vi "MVE Get Project and Library Refnums.vi"(8 "error in (no error)":errorcluster, 10 "Full Path":string) -> (0 "error out":errorcluster, 2 "ProjectItem Refnum":refnum<vi>, 3 "Project Refnum":refnum<vi>)   [LabVIEW 2016]
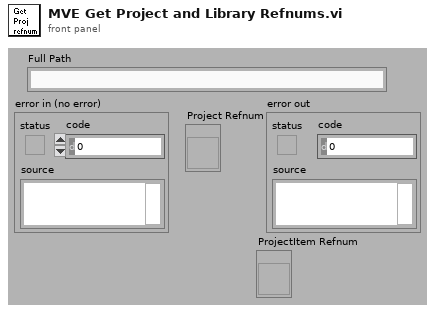
[diagram p1: front panel]
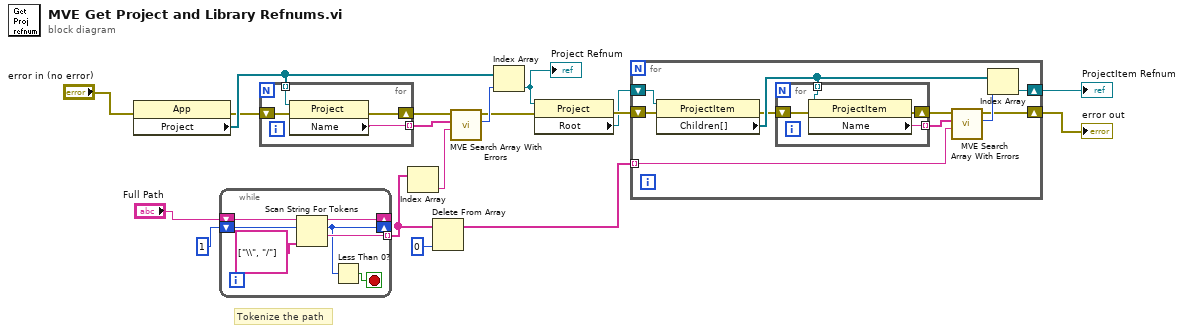
[diagram p0: block diagram]
diagram:
  # "Tokenize the path"
  n1 = property class="App"(error in="error in (no error)") -> (error out=w10:errorcluster, "Project"=w18:refnum<vi>[])  [unwired: 1 in, 1 out]
  n2 = while {
    tunnel: [w21] -> w14 mode=indexing
    shift-right: [w25] -> _
    shift-left: "Full Path" -> [w24]
    shift-right: [w19] -> _
    shift-left: 1 ("offset past token") -> [w23]
    stop <- w20 stop-if-true
    n3 = Scan String For Tokens(6:string[] ["\\", "/"] ("delimiters (\\s,\\t,\\r,\\n)"), 8:w23, 9:w24) -> (1:w21:string, 2:w19:i32, 3:w25:string)  [unwired: 3 in, 1 out]
    n4 = Less Than 0?(x=w19) -> (x < 0?=w20:bool)
  }
  n5 = for {
    tunnel: w18 -> [w29] mode=indexing
    tunnel: [w28] -> w6 mode=indexing
    shift-right: [w26] -> w7
    shift-left: w10 -> [w27]
    n6 = property class="Project"(reference=w29, error in=w27) -> (error out=w26:errorcluster, "Name"=w28:string)  [unwired: 1 out]
  }
  n7 = Index Array(array=w14) -> (element=w8:string)  [unwired: 1 in]
  n8 = Delete From Array(array=w14, index=0) -> (array with subset deleted=w5:string[])  [unwired: 1 in, 1 out]
  n9 = call <resource>:"MVE Search Array With Errors.vi"("String"=w8, "Array of Strings"=w6, "error in (no error)"=w7) -> ("index of element"=w17:i32, "error out"=w4:errorcluster)  [unwired: 7 in]
  n10 = Index Array(array=w18, index=w17) -> (element=w12:refnum<vi>)
  "Project Refnum" <- w12
  n11 = property class="Project"(reference=w12, error in=w4) -> (error out=w9:errorcluster, "Root"=w3:refnum<vi>)  [unwired: 1 out]
  n12 = for {
    tunnel: w5 -> [w32] mode=indexing
    shift-right: [w37] -> w1
    shift-left: w3 -> [w39]
    shift-right: [w33] -> w2
    shift-left: w9 -> [w35]
    n13 = property class="ProjectItem"(reference=w39, error in=w35) -> (error out=w34:errorcluster, "Children[]"=w38:refnum<vi>[])  [unwired: 1 out]
    n14 = for {
      tunnel: w38 -> [w43] mode=indexing
      tunnel: [w42] -> w31 mode=indexing
      shift-right: [w40] -> w30
      shift-left: w34 -> [w41]
      n15 = property class="ProjectItem"(reference=w43, error in=w41) -> (error out=w40:errorcluster, "Name"=w42:string)  [unwired: 1 out]
    }
    n16 = call <resource>:"MVE Search Array With Errors.vi"("String"=w32, "Array of Strings"=w31, "error in (no error)"=w30) -> ("index of element"=w36:i32, "error out"=w33:errorcluster)  [unwired: 7 in]
    n17 = Index Array(array=w38, index=w36) -> (element=w37:refnum<vi>)
  }
  "error out" <- w2
  "ProjectItem Refnum" <- w1
